vi "GetComment.vi"(8 "error in":errorcluster, 11 "UserComment in":refnum<class "UserComment.lvclass">) -> (0 "error out":errorcluster, 2 "Comment":string, 3 "UserComment out":refnum<class "UserComment.lvclass">)   [LabVIEW 2021, in "ProligentXMLGenerator.lvlib" / "UserComment.lvclass"]
uses:
  UserComment.lvclass
  UserComment.lvclass/UserComment.ctl
  Base/NonNullableString_TruncateAt_255/NonNullableString_TruncateAt_255.lvclass
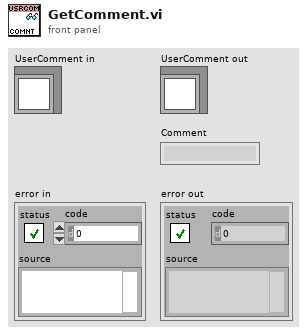
[diagram p1: front panel]
types:
  T1 = typedef "ProligentXMLGenerator.lvlib/UserComment.lvclass/Data.ctl" = cluster{"Name":string, "Comment":refnum<class "NonNullableString_TruncateAt_255.lvclass">, "User":refnum<class "NonEmptyString_255.lvclass">, "Time":refnum<class "DateTime.lvclass">}
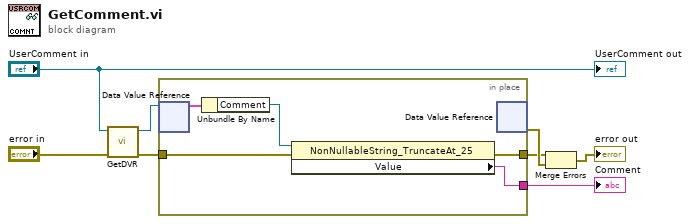
[diagram p0: block diagram]
diagram:
  n1 = call "GetDVR.vi"("error in"="error in", "UserComment"="UserComment in") -> ("error out"=w4:errorcluster, "DVRReference"=w7:refnum<data-value>)  [unwired: 8 in]
  n2 = in-place "In Place Element Structure" {
    in-place-border: w4 -> [w11]
    in-place-border: [w10] -> w3
    in-place-border: [w9] -> w1
    n3 = in-place-dvr #1(w7) -> (w13:T1)  [unwired: 1 out]
    n4 = Unbundle By Name(w13) -> ("Comment"=w12:refnum<class "NonNullableString_TruncateAt_255.lvclass">)
    n5 = property on="Property Node" class="NonNullableString_TruncateAt_25"(reference=w12, error in=w11) -> (error out=w10:errorcluster, "Value"=w9:string)  [unwired: 1 out]
    n6 = in-place-dvr #1() -> (w8:errorcluster)  [unwired: 1 in, 1 out]
  }
  "Comment" <- w1
  n7 = Merge Errors(w3, w8) -> (→"error out":errorcluster)
  "UserComment out" <- "UserComment in"
